vi "Configure Measurements Tab Source.vi"(6 "Source Count (0: 1 Source)":i32(ring) items=["1 Source", "2 Sources"], 7 "Measurement Source 2 (0: Channel 1)":i32(ring) items=["Channel 1", "Channel 2", "Channel 3", "Channel 4", "Function 1", "Function 2", "Function 3", "Function 4", "Function 5", "Function 6", "Function 7", "Function 8", "Function 9", "Function 10", "Function 11", "Function 12", "Function 13", "Function 14", "Function 15", "Function 16", "Digital 0", "Digital 1", "Digital 2", "Digital 3", "Digital 4", "Digital 5", "Digital 6", "Digital 7", "Digital 8", "Digital 9", "Digital 10", "Digital 11", "Digital 12", "Digital 13", "Digital 14", "Digital 15", "Memory 1", "Memory 2", "Memory 3", "Memory 4", "Clock", "MTRend", "MSPectrum", "Equalized"], 8 "error in (no error)":errorcluster, 9 "Measurement Source 1 (0: Channel 1)":i32(ring) items=["Channel 1", "Channel 2", "Channel 3", "Channel 4", "Function 1", "Function 2", "Function 3", "Function 4", "Function 5", "Function 6", "Function 7", "Function 8", "Function 9", "Function 10", "Function 11", "Function 12", "Function 13", "Function 14", "Function 15", "Function 16", "Digital 0", "Digital 1", "Digital 2", "Digital 3", "Digital 4", "Digital 5", "Digital 6", "Digital 7", "Digital 8", "Digital 9", "Digital 10", "Digital 11", "Digital 12", "Digital 13", "Digital 14", "Digital 15", "Memory 1", "Memory 2", "Memory 3", "Memory 4", "Clock", "MTRend", "MSPectrum", "Equalized"], 10 "Measurement Position (1: Measurement 1)":i32(ring)=1 items=["Measurement 1"=1, "Measurement 2"=2, "Measurement 3"=3, "Measurement 4"=4, "Measurement 5"=5, "Measurement 6"=6, "Measurement 7"=7, "Measurement 8"=8, "Measurement 9"=9, "Measurement 10"=10], 11 "VISA resource name":refnum<visa-resource-name>) -> (0 "error out":errorcluster, 3 "VISA resource name out":refnum<visa-resource-name>)   [LabVIEW 2013, in "Agilent 90000 Series.lvlib"]
doc: "Changes the source of an existing measurement in the Measurements tab of the user interface. Most measurement are made on the first measurement source.\n\n<b>Note:</b> This VI is new in firmware version 4.50."
uses:
  Agilent 90000 Series.lvlib
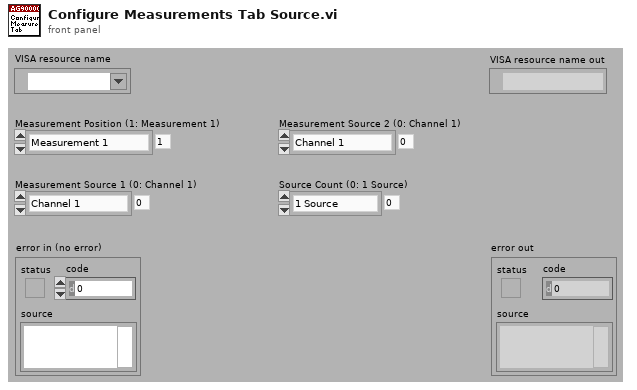
[diagram p1: front panel]
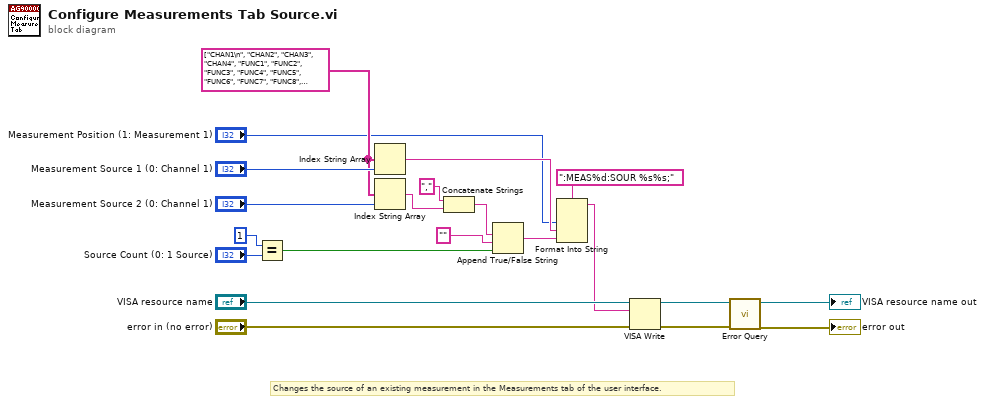
[diagram p0: block diagram]
diagram:
  w10 = string[] ["CHAN1\n", "CHAN2", "CHAN3", "CHAN4", "FUNC1", "FUNC2", "FUNC3", "FUNC4", "FUNC5", "FUNC6", "FUNC7", "FUNC8", "FUNC9", "FUNC10", "FUNC11", "FUNC12", "FUNC13", "FUNC14", "FUNC15", "FUNC16", "DIG0", "DIG1", "DIG2", "DIG3", "DIG4", "DIG5", "DIG6\n", "DIG7", "DIG8", "DIG9", "DIG10", "DIG11", "DIG12", "DIG13", "DIG14", "DIG15", "WMEM1", "WMEM2", "WMEM3", "WMEM4", "CLOC", "MTR", "MSP", "EQU"] ("subarray 2")
  # "Changes the source of an existing measurement in the Measurements tab of the user interface."
  n1 = Equal?(x=1 ("y"), y="Source Count (0: 1 Source)") -> (x = y?=w6:bool)
  n2 = Index String Array(1:"Measurement Source 1 (0: Channel 1)", 2:w10) -> (0:w9:string)  [unwired: 1 in]
  n3 = Index String Array(1:"Measurement Source 2 (0: Channel 1)", 2:w10) -> (0:w2:string)  [unwired: 1 in]
  n4 = Concatenate Strings("," ("string"), w2) -> (w4:string)
  n5 = Append True/False String(1:w6, 2:"" ("false string"), 3:w4) -> (0:w8:string)  [unwired: 1 in]
  n6 = Format Into String(format string=":MEAS%d:SOUR %s%s;", "Measurement Position (1: Measurement 1)", w9, w8) -> (resulting string=w5:string)  [unwired: 2 in, 1 out]
  n7 = VISA Write(VISA resource name="VISA resource name", write buffer=w5, error in (no error)="error in (no error)") -> (VISA resource name out=w18:refnum<visa-resource-name>, error out=w17:errorcluster)  [unwired: 1 out]
  n8 = call "Error Query.vi"("error in (no error)"=w17, "VISA resource name"=w18) -> ("error out"=→"error out":errorcluster, "VISA resource name out"=→"VISA resource name out":refnum<visa-resource-name>)  [unwired: 6 in, 2 out]
